vi "Enable Normalize Gain.vi"(8 "error in (no error)":errorcluster, 9 "Enable Normalize Gain (F: Disable)":bool, 10 "Channel Name (1: Channel 1)":i32(ring)=1 items=["Channel 1"=1, "Channel 2"=2, "Channel 3"=3, "Channel 4"=4], 11 "VISA resource name":refnum<visa-resource-name>) -> (0 "error out":errorcluster, 3 "VISA resource name out":refnum<visa-resource-name>)   [LabVIEW 2013, in "Agilent 90000 Series.lvlib"]
doc: "Activates or deactivates the \"Normalize Gain\" option.\n\n<b>Notes:</b>\n1. This Channel command only applies if you have purchased the InfiniiSim software application.\n2. This VI is new in firmware version 4.60."
uses:
  Agilent 90000 Series.lvlib
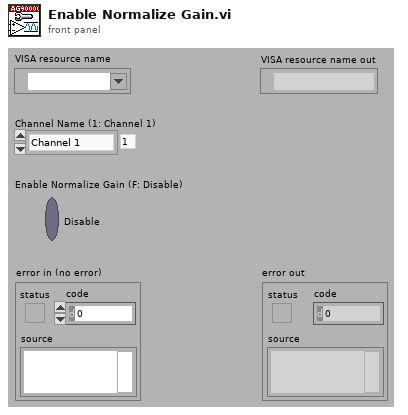
[diagram p1: front panel]
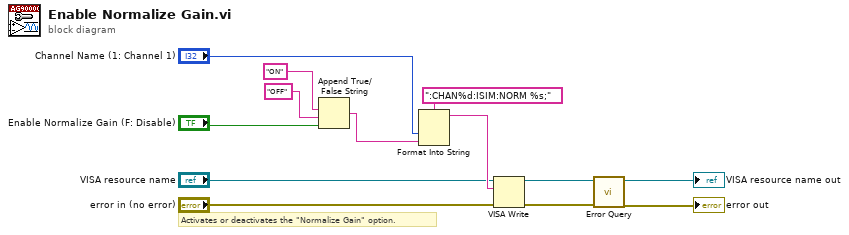
[diagram p0: block diagram]
diagram:
  # "Activates or deactivates the \"Normalize Gain\" option."
  n1 = Append True/False String(1:"Enable Normalize Gain (F: Disable)", 2:"OFF", 3:"ON") -> (0:w8:string)  [unwired: 1 in]
  n2 = Format Into String(format string=":CHAN%d:ISIM:NORM %s;", "Channel Name (1: Channel 1)", w8) -> (resulting string=w7:string)  [unwired: 2 in, 1 out]
  n3 = VISA Write(VISA resource name="VISA resource name", write buffer=w7, error in (no error)="error in (no error)") -> (VISA resource name out=w4:refnum<visa-resource-name>, error out=w3:errorcluster)  [unwired: 1 out]
  n4 = call "Error Query.vi"("error in (no error)"=w3, "VISA resource name"=w4) -> ("error out"=→"error out":errorcluster, "VISA resource name out"=→"VISA resource name out":refnum<visa-resource-name>)  [unwired: 6 in, 2 out]
